vi "Verify VI or CTL.vi"(5 "Options":T1, 7 "Test VI (caller)":string, 8 "error in":errorcluster, 9 "Extension":string, 10 "Path to Binary File to Verify":path) -> (0 "error out":errorcluster, 1 "Failure Message":string, 2 "Passed?":bool)   [LabVIEW 2020, in "Approval Tests.lvlib"]
doc: "Performs an approval test.\n\nThe first call, the test passes and the test data is written to the approved file.\n\nOn subsequent runs the test data is compared to the contents of the approved file.\nIf it is a match, the test passes.\nIf it is not a match, the test fails and the test data is written to the actual file.\n\nAt the point the user can diff the approved and actual files and determine if they approve of the changes or not. If they approve, they replace the old approved file with the actual file. \n\nNOTE: You should keep the approved files in Source Code Control. You should ignore *.actual in your .gitignore file - there is no need to store those."
uses:
  Approval Tests.lvlib
  Options.ctl
  Reporter/Reporter.lvclass
  Printer/Printer.lvclass
  <vilib>/SourceControl/sccapi/SCCAPI VI Compare Options.ctl
  <vilib>/SourceControl/sccapi/NI_SCC.lvlib
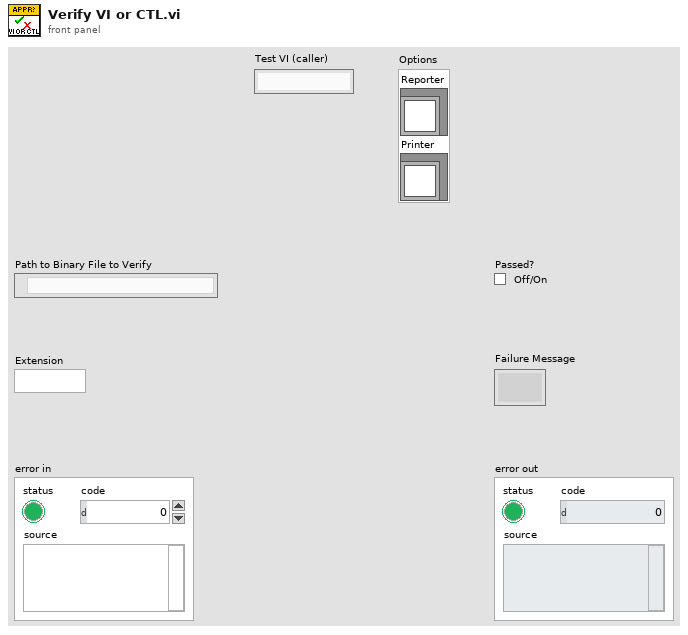
[diagram p1: front panel]
types:
  T1 = typedef "Approval Tests.lvlib/Options.ctl" = cluster{"Reporter":refnum<class "Reporter.lvclass">, "Printer":refnum<class "Printer.lvclass">}
  T2 = typedef "NI_SCC.lvlib/SCCAPI VI Compare Options.ctl" = cluster{"VI Attributes":bool, "Front Panel":bool, "FP position/size":bool, "Block Diagram":bool, "BD cosmetic":bool, "BD position/size":bool}
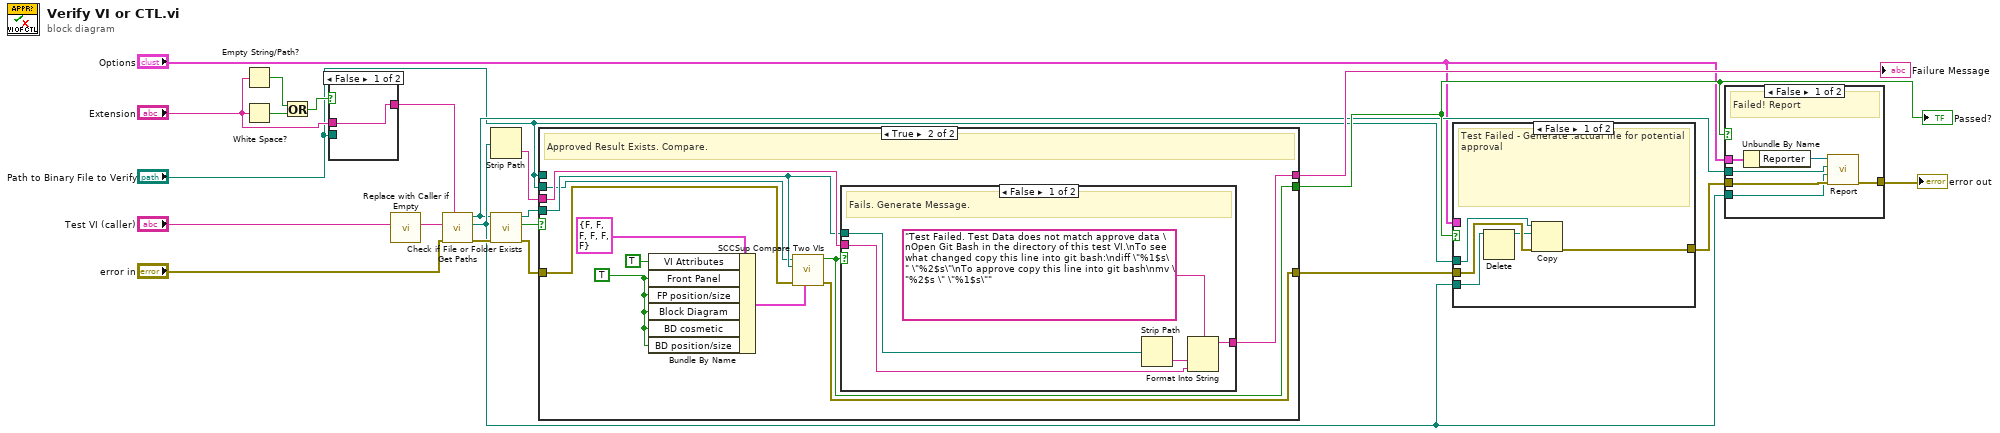
[diagram p0: block diagram]
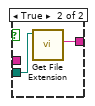
[diagram p2: hidden frame]
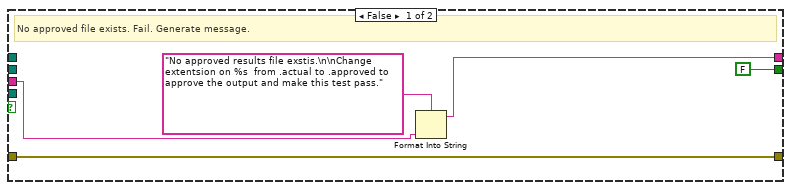
[diagram p5: hidden frame]
diagram:
  n1 = Empty String/Path?(string/path="Extension") -> (empty?=w6:bool)
  n2 = White Space?(1:"Extension") -> (0:w5:bool)
  n3 = Or(x=w6, y=w5) -> (x .or. y?=w4:bool)
  n4 = case shown="False" w4 {
    tunnel: "Path to Binary File to Verify" -> [_ w25]
    tunnel: [w23 w24] -> w3
    tunnel: "Extension" -> [w23 _]
    frame False {
    }
    frame True {
      n5 = call <vilib>:"Get File Extension.vi"("file"=w25) -> ("lowercase file extension"=w24:string)  [unwired: 6 in, 4 out]
    }
  }
  n6 = call "Replace with Caller if Empty.vi"("Test VI (caller) in"="Test VI (caller)") -> ("Test VI (caller) out"=w7:string)  [unwired: 10 in]
  n7 = call "Get Paths.vi"("Extension(txt)"=w3, "error in"="error in", "VI name"=w7) -> ("error out"=w22:errorcluster, "recived path"=w11:path, "approved path"=w10:path)  [unwired: 6 in]
  n8 = Strip Path(path=w11) -> (name=w13:string)  [unwired: 1 out]
  n9 = call <vilib>:"Check if File or Folder Exists.vi"("error in (no error)"=w22, "path"=w10) -> ("error out"=w21:errorcluster, "file or folder exists?"=w15:bool, "dup path"=w16:path)  [unwired: 7 in]
  n10 = case shown="True" w15 {
    tunnel: "Path to Binary File to Verify" -> [_ _]
    tunnel: [w30 w40] -> w20
    tunnel: w21 -> [w30 w41]
    tunnel: w16 -> [_ w36]
    tunnel: [FALSE ("Passed?") w39] -> w12
    tunnel: [w26 w38] -> w14
    tunnel: w13 -> [w28 w37]
    tunnel: "Path to Binary File to Verify" -> [_ w35]
    frame False {
      # "No approved file exists. Fail. Generate message."
      n11 = Format Into String(format string="No approved results file exstis.\n\nChange extentsion on %s  from .actual to .approved to approve the output and make this test pass.", w28) -> (resulting string=w26:string)  [unwired: 2 in, 1 out]
    }
    frame True {
      w32 = TRUE
      # "Approved Result Exists. Compare."
      n12 = Bundle By Name(cluster=T2 {"VI Attributes"=FALSE, "Front Panel"=FALSE, "FP position/size"=FALSE, "Block Diagram"=FALSE, "BD cosmetic"=FALSE, "BD position/size"=FALSE} ("compare options"), "VI Attributes"=TRUE, "Front Panel"=w32, "FP position/size"=w32, "Block Diagram"=w32, "BD cosmetic"=w32, "BD position/size"=w32) -> (w33:T2)
      n13 = call <vilib>:"SCCSup Compare Two VIs.vi"("compare options"=w33, "error in (no error)"=w41, "Second VI"=w36, "First VI"=w35) -> ("error out"=w40:errorcluster, "Same?"=w39:bool)  [unwired: 5 in, 1 out]
      n14 = case shown="False" w39 {
        tunnel: [w46 _] -> w38
        tunnel: w36 -> [w43 _]
        tunnel: w37 -> [w42 _]
        frame False {
          # "Fails. Generate Message."
          n15 = Strip Path(path=w43) -> (name=w44:string)  [unwired: 1 out]
          n16 = Format Into String(format string="Test Failed. Test Data does not match approve data \nOpen Git Bash in the directory of this test VI.\nTo see what changed copy this line into git bash:\ndiff \"%1$s\" \"%2$s\"\nTo approve copy this line into git bash\nmv \"%2$s \" \"%1$s\"", w44, w42) -> (resulting string=w46:string)  [unwired: 2 in, 1 out]
        }
        frame True {
          # "Passes. No Message Needed.."
        }
      }
    }
  }
  "Passed?" <- w12
  "Failure Message" <- w14
  n17 = case shown="False" w12 {
    tunnel: w20 -> [w51 w52]
    tunnel: [w50 w52] -> w19
    tunnel: w11 -> [w49 _]
    tunnel: "Path to Binary File to Verify" -> [w47 _]
    tunnel: "Options" -> [_ _]
    frame False {
      # "Test Failed - Generate .actual file for potential approval"
      n18 = Delete(path (use dialog)=w49) -> (deleted path=w48:path)  [unwired: 4 in, 2 out]
      n19 = Copy(8:w51, 10:w48, 11:w47) -> (0:w50:errorcluster)  [unwired: 2 in, 2 out]
    }
    frame True {
      # "Passed - no need for .actual file"
    }
  }
  n20 = case shown="False" w12 {
    tunnel: w11 -> [w55 _]
    tunnel: w10 -> [w56 _]
    tunnel: w19 -> [w58 w59]
    tunnel: [w57 w59] -> w18
    tunnel: "Options" -> [w54 _]
    frame False {
      # "Failed! Report"
      n21 = Unbundle By Name(w54) -> ("Reporter"=w53:refnum<class "Reporter.lvclass">)
      n22 = call-dynamic "Report.vi"("error in (no error)"=w58, "Received"=w55, "Approved"=w56, "Reporter in"=w53) -> ("error out"=w57:errorcluster)  [unwired: 5 in, 2 out]
    }
    frame True {
      # "Passed - Nothing to Report"
    }
  }
  "error out" <- w18
